vi "DBL Write to Buffer.vi"(8 "error in (no error)":errorcluster, 10 "Data":dbl[](array[numeric]), 11 "DBL Waveform Buffer in":refnum<class "DBL Waveform Buffer.lvclass">) -> (0 "error out":errorcluster, 3 "DBL Waveform Buffer out":refnum<class "DBL Waveform Buffer.lvclass">)   [LabVIEW 2015, in "DBL Waveform Buffer.lvclass"]
uses:
  DBL Waveform Buffer.lvclass
  Waveform Buffer/Waveform Buffer.lvclass/Waveform Buffer.ctl
  DBL Waveform Buffer.lvclass/DBL Waveform Buffer.ctl
  Waveform Buffer/Waveform Buffer.lvclass
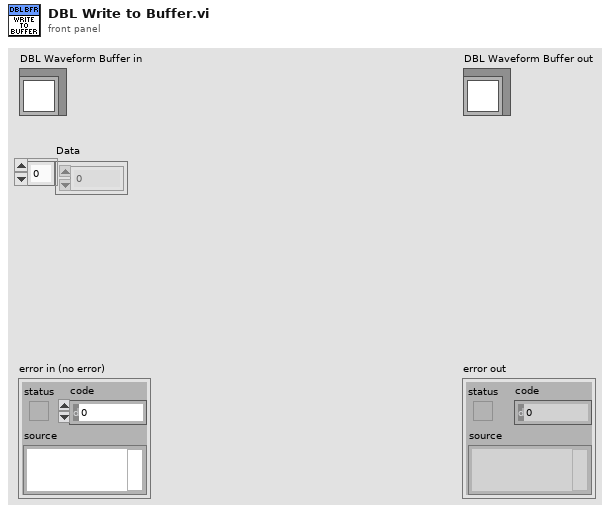
[diagram p1: front panel]
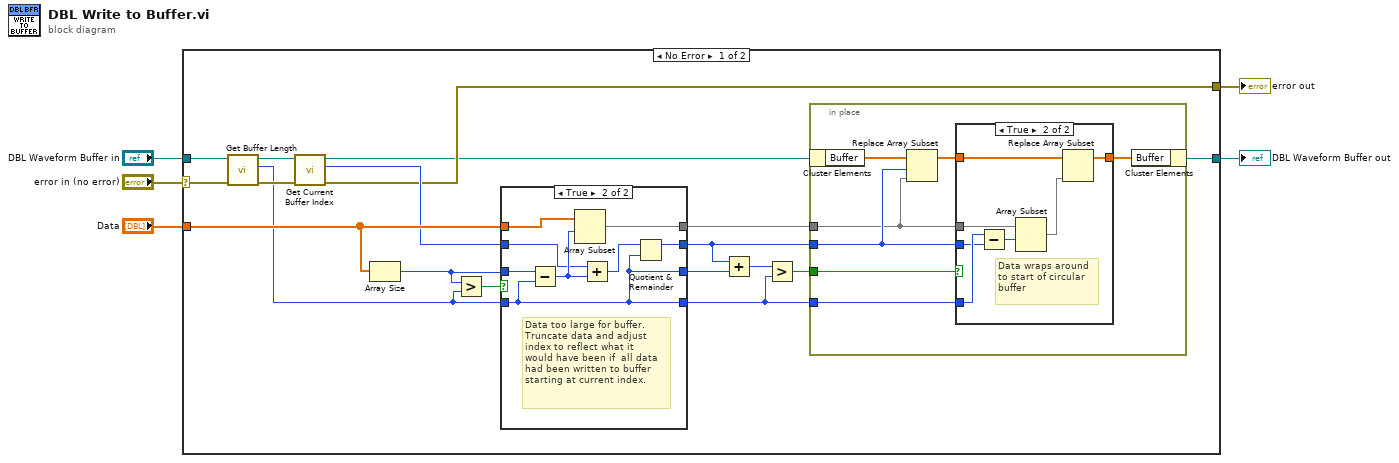
[diagram p0: block diagram]
diagram:
  n1 = case shown="No Error" "error in (no error)" {
    selector: "error in (no error)" -> [w11 w52]
    tunnel: [w7 w52] -> w4
    tunnel: [w23 w51] -> w2
    tunnel: "DBL Waveform Buffer in" -> [w12 w51]
    tunnel: "Data" -> [w18 _]
    frame No Error {
      n2 = call "Get Buffer Length.vi"("error in (no error)"=w11, "Waveform Buffer in"=w12) -> ("error out"=w10:errorcluster, "Length"=w8:i32, "Waveform Buffer out"=w9:refnum<class "DBL Waveform Buffer.lvclass">)  [unwired: 7 in]
      n3 = call "Get Current Buffer Index.vi"("error in (no error)"=w10, "Waveform Buffer in"=w9) -> ("error out"=w7:errorcluster, "Current Buffer Index"=w13:i32, "Waveform Buffer out"=w6:refnum<class "DBL Waveform Buffer.lvclass">)  [unwired: 7 in]
      n4 = Array Size(array=w18) -> (size(s)=w16:i32)
      n5 = Greater?(x=w16, y=w8) -> (0:w20:bool)
      n6 = case shown="True" w20 {
        tunnel: w18 -> [w26 w35]
        tunnel: w13 -> [w27 w31]
        tunnel: [w27 w29] -> w19
        tunnel: [w26 w34] -> w17
        tunnel: w16 -> [w25 w33]
        tunnel: w8 -> [w24 w28]
        tunnel: [w25 w28] -> w15
        tunnel: [w24 w28] -> w14
        frame False {
          # "Data will fit in buffer"
        }
        frame True {
          # "Data too large for buffer.\nTruncate data and adjust\nindex to reflect what it\nwould have been if  all data\nhad been written to buffer\nstarting at current index."
          n7 = Subtract(x=w33, y=w28) -> (x-y=w32:i32)
          n8 = Array Subset(array=w35, index=w32) -> (w34:dbl[])  [unwired: 1 in]
          n9 = Add(x=w31, y=w32) -> (x+y=w30:i32)
          n10 = Quotient & Remainder(x=w30, y=w28) -> (x-y*floor(x/y)=w29:i32)  [unwired: 1 out]
        }
      }
      n11 = Add(x=w19, y=w15) -> (x+y=w22:i32)
      n12 = Greater?(x=w22, y=w14) -> (0:w21:bool)
      n13 = in-place {
        in-place-border: w17 -> [w38]
        in-place-border: w19 -> [w39]
        in-place-border: w14 -> [w37]
        in-place-border: w21 -> [w36]
        n14 = in-place-cluster #1(w6) -> ("Buffer"=w42:dbl[])
        n15 = Replace Array Subset(array=w42, new element=w38, index=w39) -> (w41:dbl[])
        n16 = case shown="True" w36 {
          tunnel: w41 -> [w43 w50]
          tunnel: [w43 w49] -> w40
          tunnel: w38 -> [_ w48]
          tunnel: w37 -> [_ w45]
          tunnel: w39 -> [_ w44]
          frame False {
            # "Data doesn't\nwrap around"
          }
          frame True {
            # "Data wraps around\nto start of circular\nbuffer"
            n17 = Subtract(x=w45, y=w44) -> (x-y=w46:i32)
            n18 = Array Subset(array=w48, index=w46) -> (w47:dbl[])  [unwired: 1 in]
            n19 = Replace Array Subset(array=w50, new element=w47) -> (w49:dbl[])  [unwired: 1 in]
          }
        }
        n20 = in-place-cluster #1("Buffer"=w40) -> (w23:refnum<class "DBL Waveform Buffer.lvclass">)
      }
    }
    frame Error {
    }
  }
  "error out" <- w4
  "DBL Waveform Buffer out" <- w2
